vi "Feed Immediate.vi"(7 "Description":string, 8 "Command Info In":T1, 9 "Deadband Value":dbl=0.01, 10 "Lower":dbl, 11 "Upper":dbl) -> (0 "Command Info Out":T1)   [LabVIEW 2020]
doc: "This template includes code for deadband comparision to avoid excessive command scheduling. It is particularly useful for joystick-driven commands.\n\nBe sure to right-click and select New from Template and save with a new command name."
uses:
  <vilib>/Rock Robotics/WPI/Framework/Command Status Info.ctl
  <vilib>/Rock Robotics/WPI/Framework/Completion Status.ctl
  <vilib>/Rock Robotics/WPI/Framework/Completion Notifier.ctl
  Implementation/Feed Setpoints.ctl
  Implementation/Feed Operations.ctl
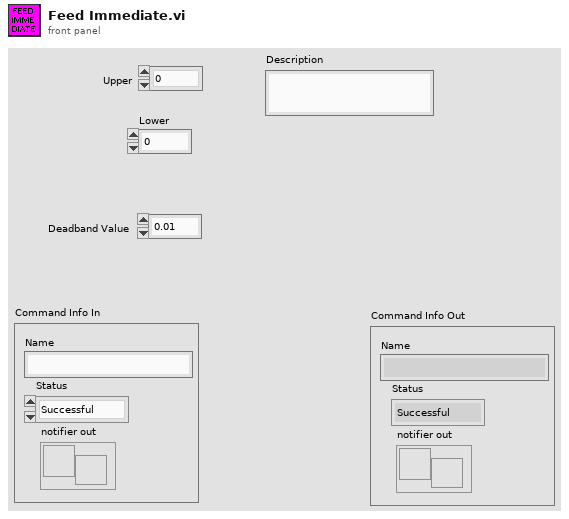
[diagram p1: front panel]
types:
  T1 = typedef "Command Status Info.ctl" = cluster{"Name":string, "Status":T2, "notifier out":T3}
  T2 = typedef "Completion Status.ctl" = enum16{"Successful", "Aborted", "Incomplete"}
  T3 = typedef "Completion Notifier.ctl" = refnum<notifier>
  T4 = typedef "Feed Setpoints.ctl" = cluster{"Operation":T5, "Upper Conveyor":dbl, "Duration":dbl, "Lower Conveyor":dbl}
  T5 = typedef "Feed Operations.ctl" = enum16{"Reserve", "Read Current", "Immediate", "Feed For Time", "Feed For Sensor"}
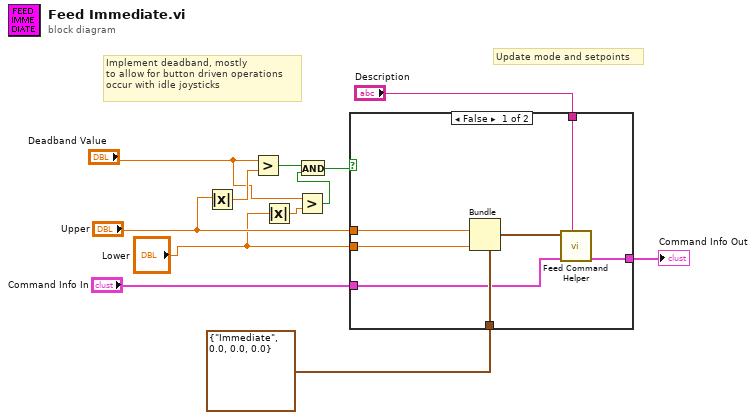
[diagram p0: block diagram]
diagram:
  # "Implement deadband, mostly\nto allow for button driven operations\noccur with idle joysticks"
  # "Update mode and setpoints"
  n1 = Absolute Value(x="Upper") -> (abs(x)=w12:dbl)
  n2 = Greater?(x="Deadband Value", y=w12) -> (0:w6:bool)
  n3 = Absolute Value(x="Lower") -> (abs(x)=w3:dbl)
  n4 = Greater?(x="Deadband Value", y=w3) -> (0:w1:bool)
  n5 = And(x=w6, y=w1) -> (x .and. y?=w5:bool)
  n6 = case shown="False" w5 {
    tunnel: "Upper" -> [w19 _]
    tunnel: T4 {"Operation"=enum."Immediate", "Upper Conveyor"=0.0, "Duration"=0.0, "Lower Conveyor"=0.0} ("SubSystem Data") -> [w18 _]
    tunnel: [w17 w20] -> w11
    tunnel: "Command Info In" -> [w16 w20]
    tunnel: "Description" -> [w14 _]
    tunnel: "Lower" -> [w13 _]
    frame False {
      n7 = Bundle(cluster=w18, "Upper Conveyor"=w19, "Lower Conveyor"=w13) -> (w15:T4)  [unwired: 2 in]
      n8 = call "Feed Command Helper.vi"("Description"=w14, "Command Info In"=w16, "SubSystem Data"=w15) -> ("Command Info Out"=w17:T1)  [unwired: 6 in, 2 out]
    }
    frame True {
    }
  }
  "Command Info Out" <- w11
